vi "Translator.GatherControls.vi"(7 "VI name":string, 8 "error in":errorcluster) -> (0 "error out":errorcluster, 2 "Controls out":T1[](array[typedef]))   [LabVIEW 2016]
uses:
  Translator.ControlData.ctl
  Translator.ControlTypes.ctl
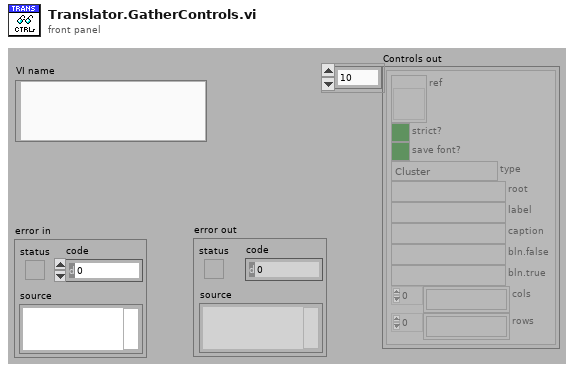
[diagram p1: front panel]
types:
  T1 = typedef "Translator.ControlData.ctl" = cluster{"ref":refnum<vi>, "strict?":bool, "save font?":bool, "type":T2, "root":string, "label":string, "caption":string, "bln.false":string, "bln.true":string, "cols":string[], "rows":string[]}
  T2 = typedef "Translator.ControlTypes.ctl" = enum16{"Cluster", "Array", "Boolean", "Ring", "String", "Tab", "Listbox", "Multicolumn listbox", "Table", "Tree", "Other"}
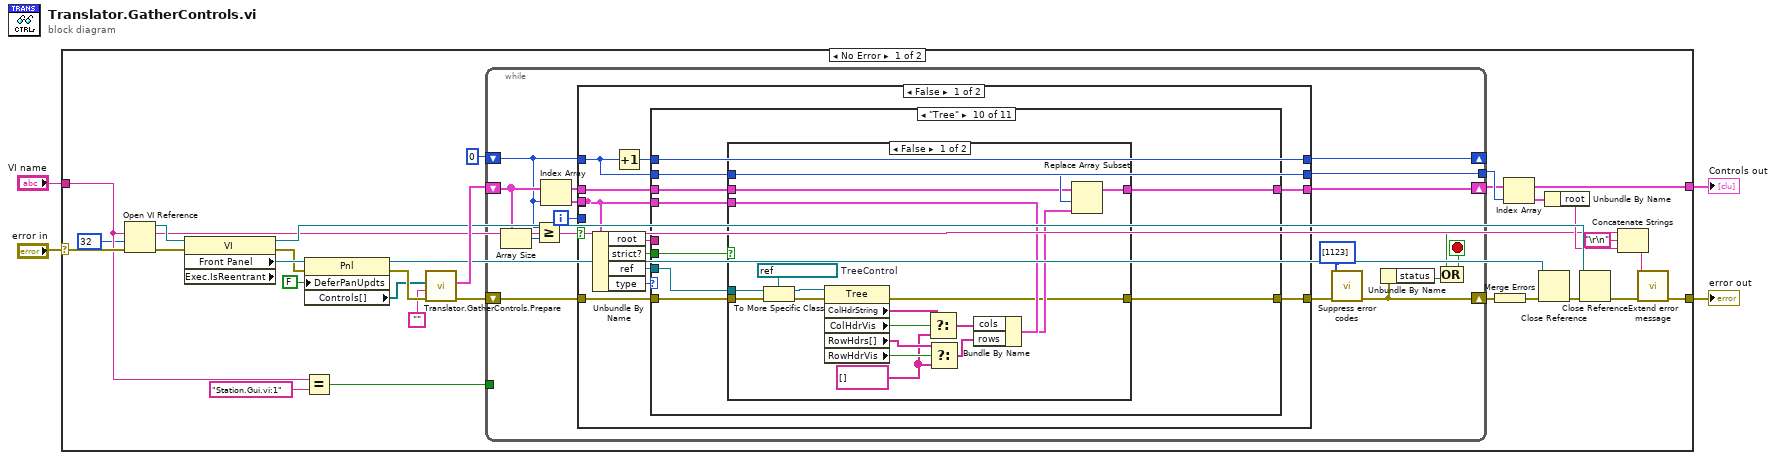
[diagram p0: block diagram]
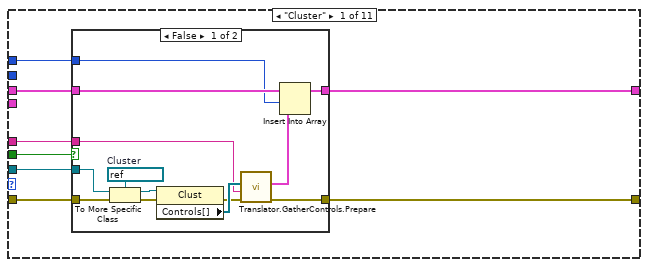
[diagram p2: hidden frame]
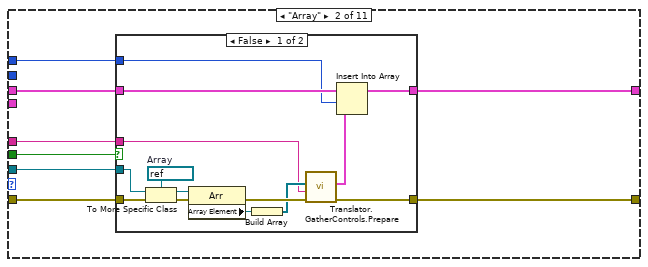
[diagram p4: hidden frame]
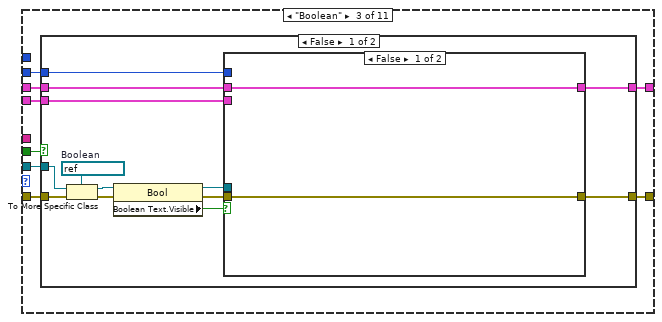
[diagram p6: hidden frame]
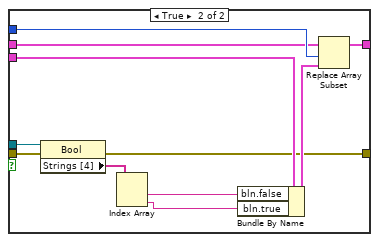
[diagram p7: hidden frame]
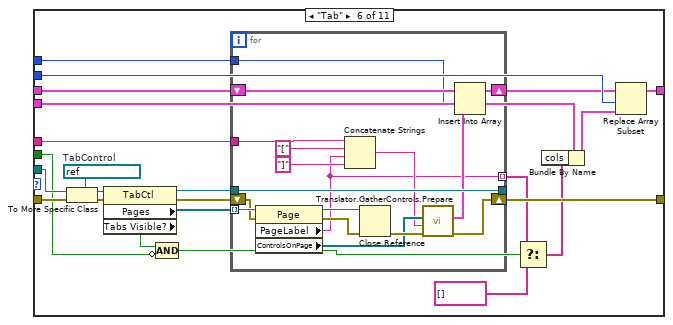
[diagram p11: hidden frame]
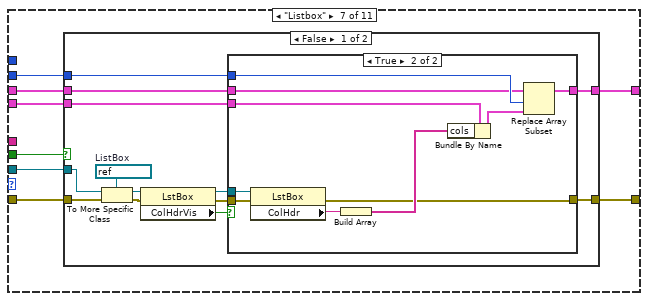
[diagram p12: hidden frame]
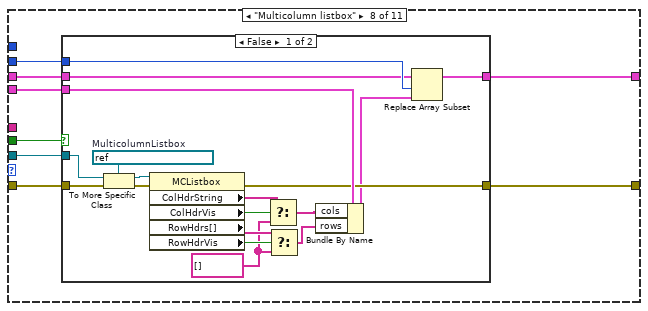
[diagram p15: hidden frame]
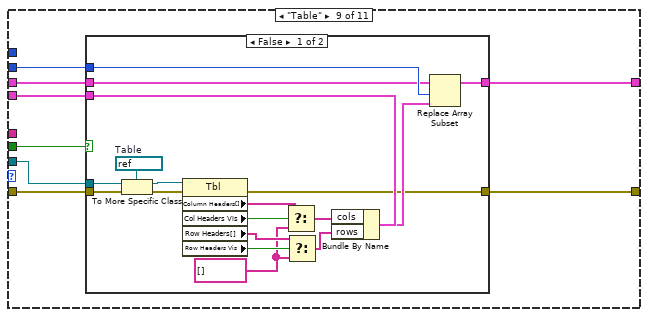
[diagram p17: hidden frame]
diagram:
  n1 = case shown="No Error" "error in" {
    selector: "error in" -> [w32 w311]
    tunnel: [w20 w311] -> w3
    tunnel: "VI name" -> [w8 _]
    tunnel: [w11 _] -> w1
    frame No Error {
      n2 = Open VI Reference(vi path=w8, options=32, error in (no error)=w32) -> (vi reference=w9:refnum<vi>, error out=w10:errorcluster)  [unwired: 3 out]
      n3 = property class="VI" props=["Front Panel", "Exec.IsReentrant"](reference=w9, error in=w10) -> (reference out=w22:refnum<vi>, error out=w31:errorcluster, "Front Panel"=w33:refnum<vi>)  [unwired: 1 out]
      n4 = Equal?(x=w8, y="Station.Gui.vi:1") -> (x = y?=w6:bool)
      n5 = property class="Pnl"(reference=w33, error in=w31, "DeferPanUpdts"=FALSE ("Defer Panel Updates")) -> (reference out=w23:refnum<vi>, error out=w27:errorcluster, "Controls[]"=w17:refnum<vi>[])
      n6 = call "Translator.GatherControls.Prepare.vi"("error in"=w27, "root"="", "Controls in"=w17) -> ("error out"=w26:errorcluster, "Controls out"=w28:T1[])  [unwired: 7 in]
      n7 = while {
        shift-right: [w44] -> w11
        shift-left: w28 -> [w45]
        shift-right: [w41] -> _
        shift-left: 0 -> [w43]
        tunnel: [w42] -> w18
        shift-right: [w37] -> w24
        shift-left: w26 -> [w46]
        tunnel: w6 -> [_]
        i -> [w34]
        stop <- w38 stop-if-true
        n8 = Array Size(array=w45) -> (size(s)=w48:i32)
        n9 = Greater Or Equal?(x=w43, y=w48) -> (x >= y?=w39:bool)
        n10 = Index Array(array=w45, index=w43) -> (element=w35:T1)
        n11 = case shown="False" w39 {
          tunnel: w35 -> [w50 _]
          tunnel: w46 -> [w57 w309]
          tunnel: w45 -> [w56 w310]
          tunnel: w43 -> [w51 w308]
          tunnel: [w49 w310] -> w44
          tunnel: [w55 w309] -> w40
          tunnel: [w51 w308] -> w42
          tunnel: [w54 w308] -> w41
          tunnel: w35 -> [_ _]
          tunnel: w34 -> [_ _]
          frame False {
            n12 = Unbundle By Name(w50) -> ("root"=w52:string, "strict?"=w53:bool, "ref"=w58:refnum<vi>, "type"=w59:T2)
            n13 = Increment(x=w51) -> (x+1=w54:i32)
            n14 = case shown="\"Tree\"" w59 {
              tunnel: w58 -> [w67 w90 w113 _ _ w163 w193 w228 w256 w284 _]
              tunnel: w57 -> [w66 w89 w114 w143 w145 w164 w194 w229 w257 w285 w306]
              tunnel: w56 -> [w65 w88 w110 w144 w146 w162 w189 w224 w252 w280 w307]
              tunnel: w54 -> [w64 w87 _ _ _ w161 _ _ _ _ _]
              tunnel: w53 -> [w60 w83 w107 _ _ w151 w187 w222 w250 w278 _]
              tunnel: w50 -> [_ _ w112 _ _ w160 w192 w227 w255 w283 _]
              tunnel: w51 -> [_ _ w111 _ _ w159 w191 w226 w254 w282 _]
              tunnel: [w63 w86 w109 w144 w146 w156 w190 w225 w253 w281 w307] -> w49
              tunnel: [w62 w85 w108 w143 w145 w155 w188 w223 w251 w279 w306] -> w55
              tunnel: w52 -> [w61 w84 _ _ _ w154 _ _ _ _ _]
              frame "Cluster" {
                n15 = case shown="False" w60 {
                  tunnel: w67 -> [w79 _]
                  tunnel: [w70 w82] -> w62
                  tunnel: w66 -> [w76 w82]
                  tunnel: w65 -> [w75 w81]
                  tunnel: [w73 w81] -> w63
                  tunnel: w64 -> [w69 _]
                  tunnel: w61 -> [w68 _]
                  frame False {
                    w80 = refnum<vi> refnum  # Cluster
                    n16 = To More Specific Class(target class=w80, reference=w79, error in=w76) -> (specific class reference=w78:refnum<vi>, error out=w77:errorcluster)
                    n17 = property class="Clust"(reference=w78, error in=w77) -> (error out=w71:errorcluster, "Controls[]"=w74:refnum<vi>[])  [unwired: 1 out]
                    n18 = call "Translator.GatherControls.Prepare.vi"("error in"=w71, "root"=w68, "Controls in"=w74) -> ("error out"=w70:errorcluster, "Controls out"=w72:T1[])  [unwired: 7 in]
                    n19 = Insert Into Array(array=w75, index=w69, new element=w72) -> (w73:T1[])
                  }
                  frame True {
                  }
                }
              }
              frame "Array" {
                n20 = case shown="False" w83 {
                  tunnel: w90 -> [w104 _]
                  tunnel: [w95 w106] -> w85
                  tunnel: w89 -> [w101 w106]
                  tunnel: w88 -> [w100 w105]
                  tunnel: [w98 w105] -> w86
                  tunnel: w87 -> [w94 _]
                  tunnel: w84 -> [w91 _]
                  frame False {
                    w93 = refnum<vi> refnum  # Array
                    n21 = To More Specific Class(target class=w93, reference=w104, error in=w101) -> (specific class reference=w103:refnum<vi>, error out=w102:errorcluster)
                    n22 = property class="Arr"(reference=w103, error in=w102) -> (error out=w96:errorcluster, "Array Element"=w99:refnum<vi>)  [unwired: 1 out]
                    n23 = Build Array(w99) -> (w92:refnum<vi>[])
                    n24 = call "Translator.GatherControls.Prepare.vi"("error in"=w96, "root"=w91, "Controls in"=w92) -> ("error out"=w95:errorcluster, "Controls out"=w97:T1[])  [unwired: 7 in]
                    n25 = Insert Into Array(array=w100, index=w94, new element=w97) -> (w98:T1[])
                  }
                  frame True {
                  }
                }
              }
              frame "Boolean" {
                n26 = case shown="False" w107 {
                  tunnel: w114 -> [w124 w141]
                  tunnel: w113 -> [w123 _]
                  tunnel: w112 -> [w122 _]
                  tunnel: w111 -> [w121 _]
                  tunnel: w110 -> [w120 w142]
                  tunnel: [w119 w142] -> w109
                  tunnel: [w115 w141] -> w108
                  frame False {
                    w127 = refnum<vi> refnum  # Boolean
                    n27 = To More Specific Class(target class=w127, reference=w123, error in=w124) -> (specific class reference=w126:refnum<vi>, error out=w125:errorcluster)
                    n28 = property class="Bool"(reference=w126, error in=w125) -> (reference out=w116:refnum<vi>, error out=w117:errorcluster, "Boolean Text.Visible"=w118:bool)
                    n29 = case shown="False" w118 {
                      tunnel: w122 -> [_ w140]
                      tunnel: w121 -> [_ w136]
                      tunnel: w120 -> [w129 w135]
                      tunnel: [w129 w134] -> w119
                      tunnel: w117 -> [w128 w133]
                      tunnel: w116 -> [_ w132]
                      tunnel: [w128 w131] -> w115
                      frame False {
                      }
                      frame True {
                        n30 = property class="Bool"(reference=w132, error in=w133) -> (error out=w131:errorcluster, "Strings [4]"=w130:string[])  [unwired: 1 out]
                        n31 = Index Array(array=w130) -> (element #1=w139:string, element #2=w138:string)  [unwired: 2 in]
                        n32 = Bundle By Name(cluster=w140, "bln.false"=w139, "bln.true"=w138) -> (w137:T1)
                        n33 = Replace Array Subset(array=w135, new element=w137, index=w136) -> (w134:T1[])
                      }
                    }
                  }
                  frame True {
                  }
                }
              }
              frame "String" {
              }
              frame "Ring" {
              }
              frame "Tab" {
                w169 = refnum<vi> refnum  # TabControl
                n34 = To More Specific Class(target class=w169, reference=w163, error in=w164) -> (specific class reference=w165:refnum<vi>, error out=w168:errorcluster)
                n35 = property class="TabCtl"(reference=w165, error in=w168) -> (reference out=w166:refnum<vi>, error out=w167:errorcluster, "Pages"=w147:refnum<vi>[], "Tabs Visible?"=w150:bool)
                n36 = Compound Arithmetic op=AND(w150, invert w151) -> (w149:bool)
                n37 = for {
                  tunnel: w147 -> [w185] mode=indexing
                  tunnel: w166 -> [w186]
                  tunnel: [w186] -> _
                  shift-right: [w175] -> w155
                  shift-left: w167 -> [w184]
                  shift-right: [w177] -> w158
                  shift-left: w162 -> [w179]
                  tunnel: w161 -> [w176]
                  tunnel: [w170] -> w153 mode=indexing
                  tunnel: w154 -> [w174]
                  n38 = property class="Page"(reference=w185, error in=w184) -> (reference out=w182:refnum<vi>, error out=w183:errorcluster, "PageLabel"=w170:string, "ControlsOnPage"=w180:refnum<vi>[])
                  n39 = Concatenate Strings(w174, "[" ("string"), w170, "]" ("string")) -> (w171:string)
                  n40 = Close Reference(reference=w182, error in (no error)=w183) -> (error out=w181:errorcluster)
                  n41 = call "Translator.GatherControls.Prepare.vi"("error in"=w181, "root"=w171, "Controls in"=w180) -> ("error out"=w175:errorcluster, "Controls out"=w178:T1[])  [unwired: 7 in]
                  n42 = Insert Into Array(array=w179, index=w176, new element=w178) -> (w177:T1[])
                }
                n43 = Select(t=w153, s=w149, f=string[] [] ("pages/legend")) -> (s? t:f=w152:string[])
                n44 = Bundle By Name(cluster=w160, "cols"=w152) -> (w157:T1)
                n45 = Replace Array Subset(array=w158, new element=w157, index=w159) -> (w156:T1[])
              }
              frame "Listbox" {
                n46 = case shown="False" w187 {
                  tunnel: w194 -> [w204 w221]
                  tunnel: w193 -> [w203 _]
                  tunnel: w192 -> [w202 _]
                  tunnel: w191 -> [w201 _]
                  tunnel: [w200 w220] -> w190
                  tunnel: w189 -> [w199 w220]
                  tunnel: [w196 w221] -> w188
                  frame False {
                    w207 = refnum<vi> refnum  # ListBox
                    n47 = To More Specific Class(target class=w207, reference=w203, error in=w204) -> (specific class reference=w205:refnum<vi>, error out=w206:errorcluster)
                    n48 = property class="LstBox"(reference=w205, error in=w206) -> (reference out=w197:refnum<vi>, error out=w195:errorcluster, "ColHdrVis"=w198:bool)
                    n49 = case shown="True" w198 {
                      tunnel: w202 -> [_ w216]
                      tunnel: w201 -> [_ w219]
                      tunnel: [w208 w218] -> w200
                      tunnel: w199 -> [w208 w217]
                      tunnel: w195 -> [w209 w213]
                      tunnel: w197 -> [_ w212]
                      tunnel: [w209 w210] -> w196
                      frame False {
                      }
                      frame True {
                        n50 = property class="LstBox"(reference=w212, error in=w213) -> (error out=w210:errorcluster, "ColHdr"=w214:string)  [unwired: 1 out]
                        n51 = Build Array(w214) -> (w211:string[])
                        n52 = Bundle By Name(cluster=w216, "cols"=w211) -> (w215:T1)
                        n53 = Replace Array Subset(array=w217, new element=w215, index=w219) -> (w218:T1[])
                      }
                    }
                  }
                  frame True {
                  }
                }
              }
              frame "Multicolumn listbox" {
                n54 = case shown="False" w222 {
                  tunnel: w229 -> [w244 w248]
                  tunnel: w228 -> [w243 _]
                  tunnel: w227 -> [w242 _]
                  tunnel: w226 -> [w241 _]
                  tunnel: [w240 w249] -> w225
                  tunnel: w224 -> [w238 w249]
                  tunnel: [w237 w248] -> w223
                  frame False {
                    w233 = string[] [] ("f")
                    w247 = refnum<vi> refnum  # MulticolumnListbox
                    n55 = To More Specific Class(target class=w247, reference=w243, error in=w244) -> (specific class reference=w245:refnum<vi>, error out=w246:errorcluster)
                    n56 = property class="MCListbox"(reference=w245, error in=w246) -> (error out=w237:errorcluster, "ColHdrString"=w236:string[], "ColHdrVis"=w239:bool, "RowHdrs[]"=w234:string[], "RowHdrVis"=w235:bool)  [unwired: 1 out]
                    n57 = Select(t=w236, s=w239, f=w233) -> (s? t:f=w232:string[])
                    n58 = Select(t=w234, s=w235, f=w233) -> (s? t:f=w231:string[])
                    n59 = Bundle By Name(cluster=w242, "cols"=w232, "rows"=w231) -> (w230:T1)
                    n60 = Replace Array Subset(array=w238, new element=w230, index=w241) -> (w240:T1[])
                  }
                  frame True {
                  }
                }
              }
              frame "Table" {
                n61 = case shown="False" w250 {
                  tunnel: w257 -> [w272 w276]
                  tunnel: w256 -> [w271 _]
                  tunnel: w255 -> [w270 _]
                  tunnel: w254 -> [w269 _]
                  tunnel: [w267 w277] -> w253
                  tunnel: w252 -> [w265 w277]
                  tunnel: [w264 w276] -> w251
                  frame False {
                    w260 = string[] [] ("f")
                    w275 = refnum<vi> refnum  # Table
                    n62 = To More Specific Class(target class=w275, reference=w271, error in=w272) -> (specific class reference=w273:refnum<vi>, error out=w274:errorcluster)
                    n63 = property class="Tbl"(reference=w273, error in=w274) -> (error out=w264:errorcluster, "Column Headers[]"=w263:string[], "Col Headers Vis"=w266:bool, "Row Headers[]"=w261:string[], "Row Headers Vis"=w262:bool)  [unwired: 1 out]
                    n64 = Select(t=w263, s=w266, f=w260) -> (s? t:f=w259:string[])
                    n65 = Select(t=w261, s=w262, f=w260) -> (s? t:f=w258:string[])
                    n66 = Bundle By Name(cluster=w270, "cols"=w259, "rows"=w258) -> (w268:T1)
                    n67 = Replace Array Subset(array=w265, new element=w268, index=w269) -> (w267:T1[])
                  }
                  frame True {
                  }
                }
              }
              frame "Tree" {
                n68 = case shown="False" w278 {
                  tunnel: w285 -> [w300 w304]
                  tunnel: w284 -> [w299 _]
                  tunnel: w283 -> [w298 _]
                  tunnel: w282 -> [w297 _]
                  tunnel: [w295 w305] -> w281
                  tunnel: w280 -> [w293 w305]
                  tunnel: [w292 w304] -> w279
                  frame False {
                    w288 = string[] [] ("f")
                    w303 = refnum<vi> refnum  # TreeControl
                    n69 = To More Specific Class(target class=w303, reference=w299, error in=w300) -> (specific class reference=w301:refnum<vi>, error out=w302:errorcluster)
                    n70 = property class="Tree"(reference=w301, error in=w302) -> (error out=w292:errorcluster, "ColHdrString"=w291:string[], "ColHdrVis"=w294:bool, "RowHdrs[]"=w289:string[], "RowHdrVis"=w290:bool)  [unwired: 1 out]
                    n71 = Select(t=w291, s=w294, f=w288) -> (s? t:f=w287:string[])
                    n72 = Select(t=w289, s=w290, f=w288) -> (s? t:f=w286:string[])
                    n73 = Bundle By Name(cluster=w298, "cols"=w287, "rows"=w286) -> (w296:T1)
                    n74 = Replace Array Subset(array=w293, new element=w296, index=w297) -> (w295:T1[])
                  }
                  frame True {
                  }
                }
              }
              frame "Other" {
              }
            }
          }
          frame True {
          }
        }
        n75 = call "Suppress error codes.vi"("error in (no error)"=w40, "suppress codes([43])"=i32[] [1123]) -> ("error out"=w37:errorcluster)  [unwired: 8 in, 1 out]
        n76 = Unbundle By Name(w37) -> ("status"=w47:bool)
        n77 = Compound Arithmetic op=OR(w39, w47) -> (w38:bool)
      }
      n78 = Merge Errors(w24) -> (w13:errorcluster)
      n79 = Index Array(array=w11, index=w18) -> (element=w19:T1)
      n80 = Close Reference(reference=w23, error in (no error)=w13) -> (error out=w30:errorcluster)
      n81 = Unbundle By Name(w19) -> ("root"=w12:string)
      n82 = Close Reference(reference=w22, error in (no error)=w30) -> (error out=w21:errorcluster)
      n83 = Concatenate Strings(w8, "\r\n", w12) -> (w14:string)
      n84 = call "Extend error message.vi"("error in"=w21, "extra message part"=w14) -> ("error out"=w20:errorcluster)  [unwired: 9 in]
    }
    frame Error {
    }
  }
  "error out" <- w3
  "Controls out" <- w1
